vi "_script_fix_Parse State Queue in Find Parse State Queue vi name2.vi"   [LabVIEW 2014]
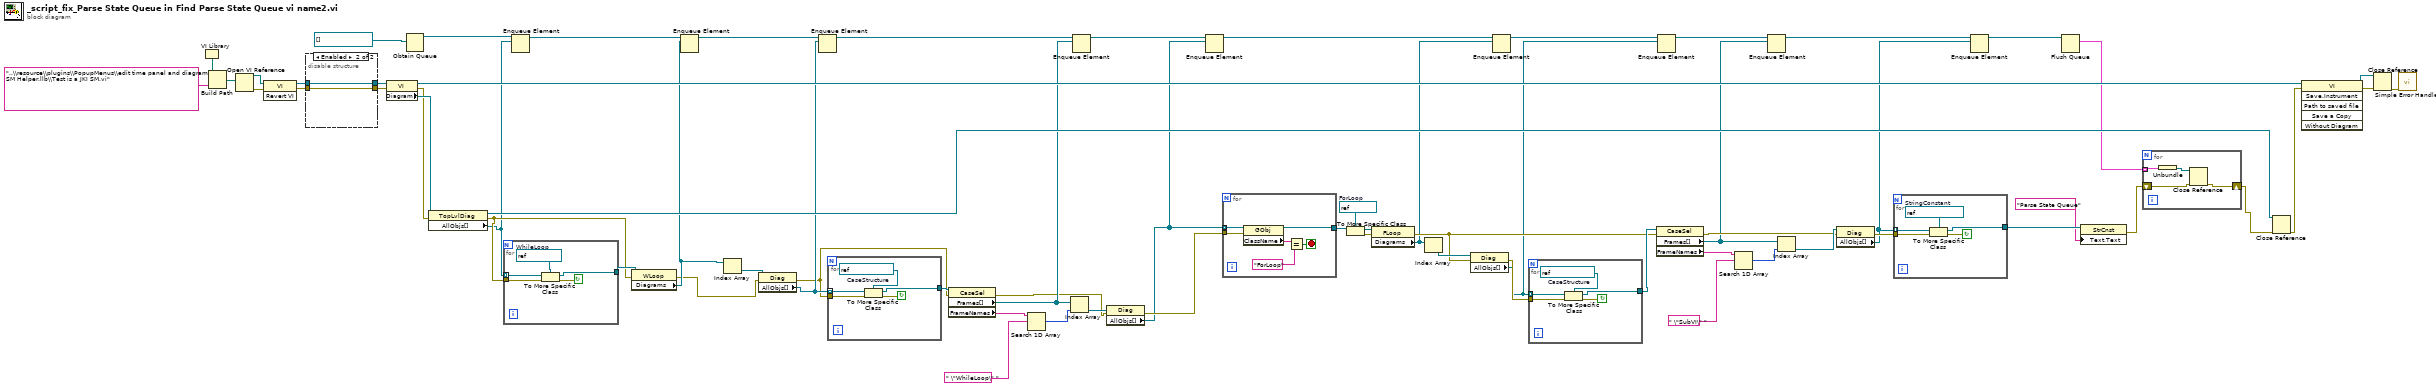
[diagram p0: block diagram]
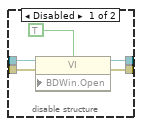
[diagram p2: hidden frame]
diagram:
  w56 = refnum<vi> refnum  # ForLoop
  n1 = VI Library() -> (path=w66:path)
  n2 = Build Path(base path=w66, name or relative path="..\\resource\\plugins\\PopupMenus\\edit time panel and diagram\\JKI SM Helper.llb\\Test is a JKI SM.vi") -> (appended path=w64:path)
  n3 = Open VI Reference(vi path=w64) -> (vi reference=w67:refnum<vi>, error out=w68:errorcluster)  [unwired: 5 in]
  n4 = invoke class="VI" method="Revert VI"(reference=w67, error in=w68) -> (reference out=w48:refnum<vi>, error out=w47:errorcluster)  [unwired: 1 in, 1 out]
  n5 = disable-structure shown="Enabled" {
    disable-tunnel: w48 -> [w73 w75]
    disable-tunnel: w47 -> [w72 w74]
    disable-tunnel: [w71 w75] -> w46
    disable-tunnel: [w70 w74] -> w45
    frame Disabled {
      n6 = property class="VI"(reference=w73, error in=w72, "BDWin.Open"=TRUE ("Block Diagram Window:Open")) -> (reference out=w71:refnum<vi>, error out=w70:errorcluster)
    }
    frame Enabled {
    }
  }
  n7 = property class="VI"(reference=w46, error in=w45) -> (reference out=w63:refnum<vi>, error out=w58:errorcluster, "Diagram"=w59:refnum<vi>)
  n8 = Obtain Queue(element data type=refnum<vi>[] [] ("All Objects[]")) -> (queue out=w32:refnum<queue>)  [unwired: 4 in, 2 out]
  n9 = property class="TopLvlDiag"(reference=w59, error in=w58) -> (reference out=w50:refnum<vi>, error out=w34:errorcluster, "AllObjs[]"=w31:refnum<vi>[])
  n10 = for {
    tunnel: w31 -> [w80] mode=indexing
    tunnel: w34 -> [w79]
    tunnel: [w77] -> w35
    stop <- w78 continue-if-true
    w76 = refnum<vi> refnum  # WhileLoop
    n11 = To More Specific Class(target class=w76, reference=w80, error in=w79) -> (specific class reference=w77:refnum<vi>, error out=w78:errorcluster)
  }
  n12 = Enqueue Element(queue=w32, element=w31) -> (queue out=w30:refnum<queue>)  [unwired: 2 in, 2 out]
  n13 = property class="WLoop"(reference=w35, error in=w34) -> (error out=w27:errorcluster, "Diagrams"=w29:refnum<vi>[])  [unwired: 1 out]
  n14 = Enqueue Element(queue=w30, element=w29) -> (queue out=w25:refnum<queue>)  [unwired: 2 in, 2 out]
  n15 = Index Array(array=w29) -> (element=w28:refnum<vi>)  [unwired: 1 in]
  n16 = property class="Diag"(reference=w28, error in=w27) -> (error out=w18:errorcluster, "AllObjs[]"=w26:refnum<vi>[])  [unwired: 1 out]
  n17 = Enqueue Element(queue=w25, element=w26) -> (queue out=w20:refnum<queue>)  [unwired: 2 in, 2 out]
  n18 = for {
    tunnel: w26 -> [w85] mode=indexing
    tunnel: w18 -> [w84]
    tunnel: [w82] -> w21
    stop <- w83 continue-if-true
    w81 = refnum<vi> refnum  # CaseStructure
    n19 = To More Specific Class(target class=w81, reference=w85, error in=w84) -> (specific class reference=w82:refnum<vi>, error out=w83:errorcluster)
  }
  n20 = property class="CaseSel"(reference=w21, error in=w18) -> (error out=w16:errorcluster, "Frames[]"=w19:refnum<vi>[], "FrameNames"=w22:string[])  [unwired: 1 out]
  n21 = Search 1D Array(1D array=w22, element=" \"WhileLoop\" " ("y")) -> (index of element=w24:i32)  [unwired: 1 in]
  n22 = Index Array(array=w19, index=w24) -> (element=w17:refnum<vi>)
  n23 = Enqueue Element(queue=w20, element=w19) -> (queue out=w13:refnum<queue>)  [unwired: 2 in, 2 out]
  n24 = property class="Diag"(reference=w17, error in=w16) -> (error out=w15:errorcluster, "AllObjs[]"=w14:refnum<vi>[])  [unwired: 1 out]
  n25 = Enqueue Element(queue=w13, element=w14) -> (queue out=w11:refnum<queue>)  [unwired: 2 in, 2 out]
  n26 = for {
    tunnel: w14 -> [w91] mode=indexing
    tunnel: w15 -> [w90]
    tunnel: [w89] -> w57
    stop <- w86 stop-if-true
    n27 = property class="GObj"(reference=w91, error in=w90) -> (reference out=w89:refnum<vi>, "ClassName"=w88:string)  [unwired: 1 out]
    n28 = Equal?(x=w88, y="ForLoop") -> (x = y?=w86:bool)
  }
  n29 = To More Specific Class(target class=w56, reference=w57) -> (specific class reference=w55:refnum<vi>, error out=w54:errorcluster)  [unwired: 1 in]
  n30 = property class="FLoop"(reference=w55, error in=w54) -> (error out=w41:errorcluster, "Diagrams"=w12:refnum<vi>[])  [unwired: 1 out]
  n31 = Index Array(array=w12) -> (element=w44:refnum<vi>)  [unwired: 1 in]
  n32 = property class="Diag"(reference=w44, error in=w41) -> (error out=w43:errorcluster, "AllObjs[]"=w9:refnum<vi>[])  [unwired: 1 out]
  n33 = Enqueue Element(queue=w11, element=w12) -> (queue out=w10:refnum<queue>)  [unwired: 2 in, 2 out]
  n34 = for {
    tunnel: w9 -> [w96] mode=indexing
    tunnel: w43 -> [w95]
    tunnel: [w93] -> w42
    stop <- w94 continue-if-true
    w92 = refnum<vi> refnum  # CaseStructure
    n35 = To More Specific Class(target class=w92, reference=w96, error in=w95) -> (specific class reference=w93:refnum<vi>, error out=w94:errorcluster)
  }
  n36 = property class="CaseSel"(reference=w42, error in=w41) -> (error out=w36:errorcluster, "Frames[]"=w8:refnum<vi>[], "FrameNames"=w40:string[])  [unwired: 1 out]
  n37 = Enqueue Element(queue=w10, element=w9) -> (queue out=w7:refnum<queue>)  [unwired: 2 in, 2 out]
  n38 = Search 1D Array(1D array=w40, element=" \"SubVI\" " ("y")) -> (index of element=w38:i32)  [unwired: 1 in]
  n39 = Enqueue Element(queue=w7, element=w8) -> (queue out=w6:refnum<queue>)  [unwired: 2 in, 2 out]
  n40 = Index Array(array=w8, index=w38) -> (element=w37:refnum<vi>)
  n41 = property class="Diag"(reference=w37, error in=w36) -> (error out=w53:errorcluster, "AllObjs[]"=w5:refnum<vi>[])  [unwired: 1 out]
  n42 = for {
    tunnel: w5 -> [w101] mode=indexing
    tunnel: w53 -> [w100]
    tunnel: [w97] -> w52
    stop <- w98 continue-if-true
    w99 = refnum<vi> refnum  # StringConstant
    n43 = To More Specific Class(target class=w99, reference=w101, error in=w100) -> (specific class reference=w97:refnum<vi>, error out=w98:errorcluster)
  }
  n44 = Enqueue Element(queue=w6, element=w5) -> (queue out=w4:refnum<queue>)  [unwired: 2 in, 2 out]
  n45 = Flush Queue(queue=w4) -> (remaining elements=w3:cluster{"All Objects[]":refnum<vi>[]}[])  [unwired: 1 in, 2 out]
  n46 = property class="StrCnst"(reference=w52, "Text.Text"="Parse State Queue") -> (error out=w2:errorcluster)  [unwired: 1 in, 1 out]
  n47 = for {
    tunnel: w3 -> [w105] mode=indexing
    shift-right: [w102] -> w1
    shift-left: w2 -> [w103]
    n48 = Unbundle(w105) -> ("All Objects[]"=w104:refnum<vi>[])
    n49 = Close Reference(reference=w104, error in (no error)=w103) -> (error out=w102:errorcluster)
  }
  n50 = Close Reference(reference=w50, error in (no error)=w1) -> (error out=w49:errorcluster)
  n51 = invoke class="VI" method="Save.Instrument"(reference=w63, error in=w49) -> (reference out=w61:refnum<vi>, error out=w62:errorcluster)  [unwired: 4 in, 4 out]
  n52 = Close Reference(reference=w61, error in (no error)=w62) -> (error out=w60:errorcluster)
  n53 = call <vilib>:"Simple Error Handler.vi"("error in (no error)"=w60) -> ()  [unwired: 4 in, 5 out]
